vi "Main.vi"() -> ()   [LabVIEW 2016]
uses:
  VI Reference Control/VI Reference Control.lvclass
panel:
  in  "Execute Script":bool
  in  "Target Path":path
  out "Target Picture":picture
  in  "Source Path":path
  out "Source Picture":picture
  in  "stop":bool
  # "Drag Target VI Here"
  # "Drag Source VI Here"
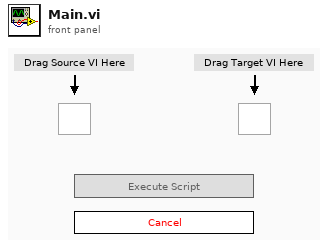
[diagram p1: front panel]
types:
  T1 = enum8{"Enabled", "Disabled", "Disabled and Grayed Out"}
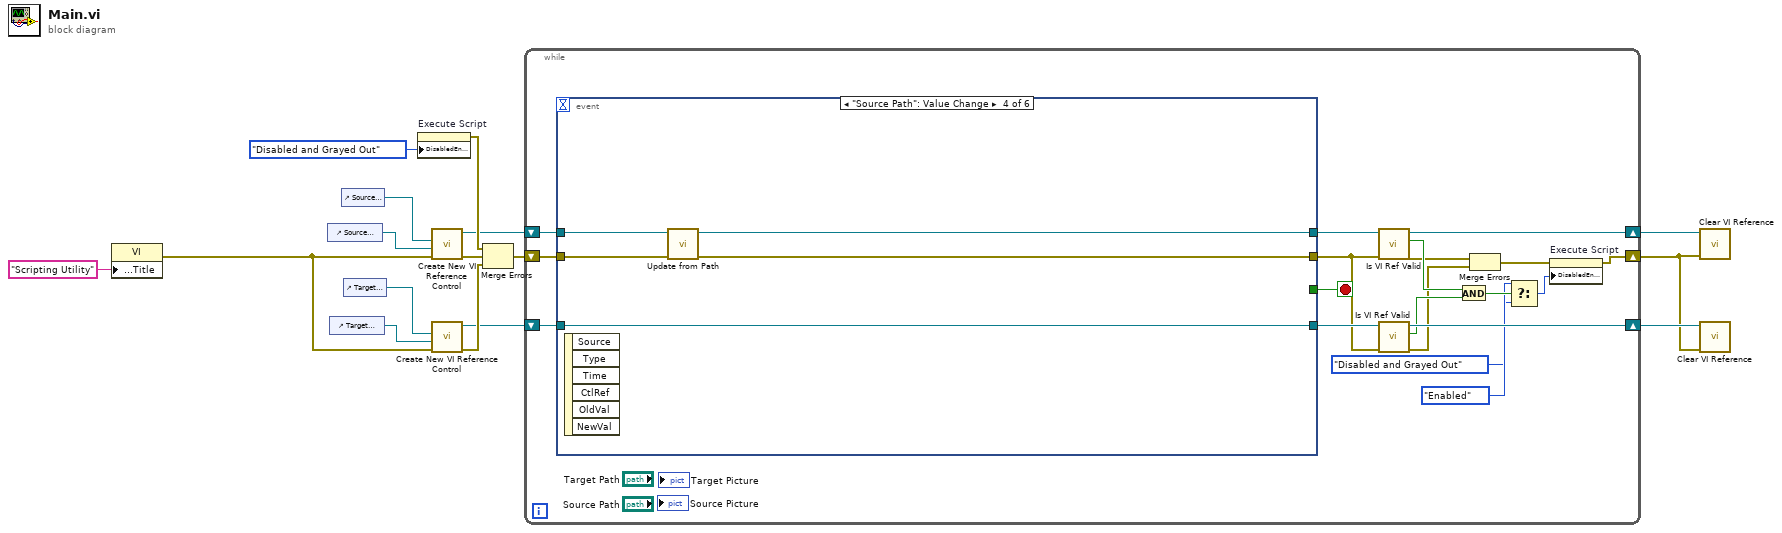
[diagram p0: block diagram]
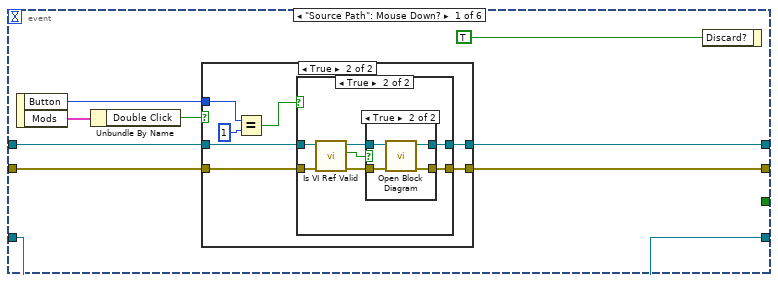
[diagram p2: hidden frame]
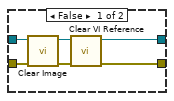
[diagram p4: hidden frame]
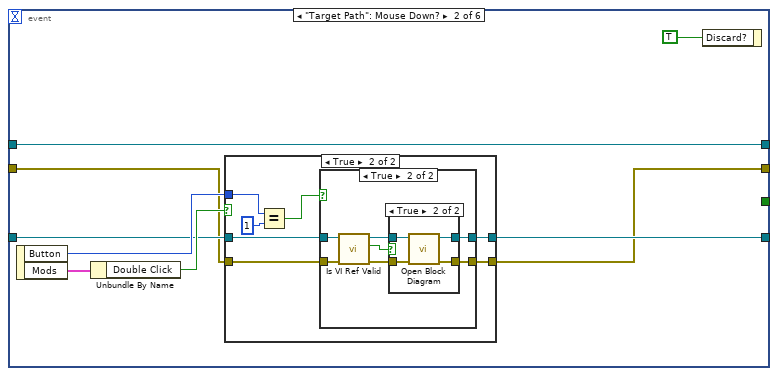
[diagram p6: hidden frame]
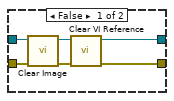
[diagram p8: hidden frame]
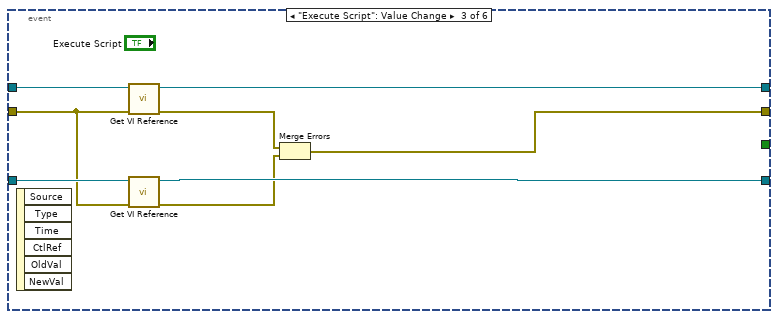
[diagram p10: hidden frame]
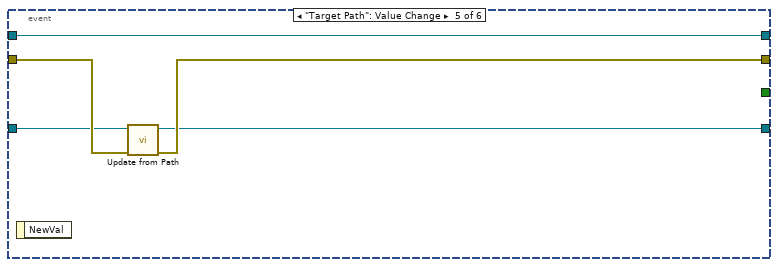
[diagram p11: hidden frame]
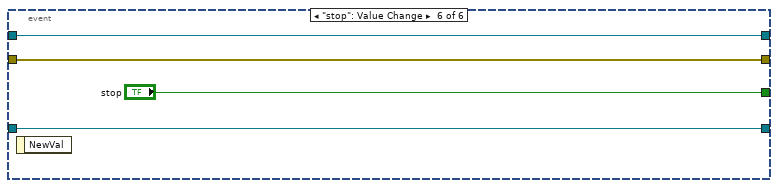
[diagram p12: hidden frame]
diagram:
  n1 = property class="VI"("Front Panel.Title"="Scripting Utility" ("Front Panel Window:Title")) -> (error out=w1:errorcluster)  [unwired: 2 in, 1 out]
  n2 = control-ref of="Source Picture"() -> (w12:refnum<vi>)
  n3 = control-ref of="Target Picture"() -> (w9:refnum<vi>)
  n4 = control-ref of="Source Path"() -> (w13:refnum<vi>)
  n5 = control-ref of="Target Path"() -> (w10:refnum<vi>)
  n6 = property on="Execute Script" class="Bool"("DisabledEnum"=T1."Disabled and Grayed Out" ("Disabled")) -> (error out=w15:errorcluster)  [unwired: 2 in, 1 out]
  n7 = call "Create New VI Reference Control.vi"("error in (no error)"=w1, "Picture Control Ref"=w12, "Path Control Ref"=w13) -> ("error out"=w8:errorcluster, "VI Reference Control out"=w11:refnum<class "VI Reference Control.lvclass">)  [unwired: 7 in]
  n8 = call "Create New VI Reference Control.vi"("error in (no error)"=w1, "Picture Control Ref"=w9, "Path Control Ref"=w10) -> ("error out"=w7:errorcluster, "VI Reference Control out"=w6:refnum<class "VI Reference Control.lvclass">)  [unwired: 7 in]
  n9 = Merge Errors(w15, w8, w7) -> (w14:errorcluster)
  n10 = while {
    shift-right: [w31] -> w3
    shift-left: w14 -> [w32]
    shift-right: [w28] -> w5
    shift-left: w11 -> [w30]
    shift-right: [w27] -> w4
    shift-left: w6 -> [w26]
    stop <- w35 stop-if-true
    n11 = event shown="[3] \"Source Path\": Value Change" {
      selector: _ -> [_ _ _ _ _ _]
      dyn-events: _ -> [_ _ _ _ _ _]
      timeout: _ -> [_ _ _ _ _ _]
      tunnel: [_ _ _ _ _ "stop"] -> w35
      tunnel: w32 -> [w40 w75 w113 w121 w127 w130]
      tunnel: [w39 w73 w110 w118 w126 w130] -> w24
      tunnel: w30 -> [w38 w79 w115 w122 w123 w129]
      tunnel: [w37 w79 w114 w120 w123 w129] -> w29
      tunnel: w26 -> [w36 w76 w117 w119 w125 w128]
      tunnel: [w36 w74 w116 w119 w124 w128] -> w25
      event "Source Path": Mouse Down? {
        n12 = event-data() -> ("Button"=w41:u16, "Mods"=w43:cluster{"Double Click":bool, "Menu Key":bool})  [unwired: 1 in]
        n13 = Unbundle By Name(w43) -> ("Double Click"=w42:bool)
        n14 = case shown="True" w42 {
          tunnel: w41 -> [_ w51]
          tunnel: w40 -> [w46 w50]
          tunnel: [w46 w49] -> w39
          tunnel: w38 -> [w45 w48]
          tunnel: [w45 w47] -> w37
          frame False {
          }
          frame True {
            n15 = Equal?(x=w51, y=u16 1) -> (x = y?=w52:bool)
            n16 = case shown="True" w52 {
              tunnel: w50 -> [w56 w61]
              tunnel: [w54 w66] -> w49
              tunnel: w48 -> [w58 w64]
              tunnel: [w59 w65] -> w47
              frame False {
                n17 = call "Clear Image.vi"("error in (no error)"=w56, "VI Reference Control in"=w58) -> ("error out"=w55:errorcluster, "VI Reference Control out"=w57:refnum<class "VI Reference Control.lvclass">)  [unwired: 8 in]
                n18 = call "Clear VI Reference.vi"("error in (no error)"=w55, "VI Reference Control in"=w57) -> ("error out"=w54:errorcluster, "VI Reference Control out"=w59:refnum<class "VI Reference Control.lvclass">)  [unwired: 8 in]
              }
              frame True {
                n19 = call "Is VI Ref Valid"("error in (no error)"=w61, "VI Reference Control in"=w64) -> ("error out"=w60:errorcluster, "Refnum Valid?"=w63:bool, "VI Reference Control out"=w62:refnum<class "VI Reference Control.lvclass">)  [unwired: 7 in]
                n20 = case shown="True" w63 {
                  tunnel: w60 -> [w68 w71]
                  tunnel: [w68 w70] -> w66
                  tunnel: w62 -> [w67 w72]
                  tunnel: [w67 w69] -> w65
                  frame False {
                  }
                  frame True {
                    n21 = call "Open Block Diagram.vi"("error in (no error)"=w71, "VI Reference Control in"=w72) -> ("error out"=w70:errorcluster, "VI Reference Control out"=w69:refnum<class "VI Reference Control.lvclass">)  [unwired: 8 in]
                  }
                }
              }
            }
          }
        }
        n22 = event-data("Discard?"=TRUE) -> ()  [unwired: 1 in, 1 out]
      }
      event "Target Path": Mouse Down? {
        n23 = event-data() -> ("Button"=w77:u16, "Mods"=w80:cluster{"Double Click":bool, "Menu Key":bool})  [unwired: 1 in]
        n24 = Unbundle By Name(w80) -> ("Double Click"=w78:bool)
        n25 = case shown="True" w78 {
          tunnel: w77 -> [_ w88]
          tunnel: w75 -> [w83 w87]
          tunnel: [w83 w86] -> w73
          tunnel: w76 -> [w82 w85]
          tunnel: [w82 w84] -> w74
          frame False {
          }
          frame True {
            n26 = Equal?(x=w88, y=u16 1) -> (x = y?=w89:bool)
            n27 = case shown="True" w89 {
              tunnel: w87 -> [w93 w98]
              tunnel: [w91 w103] -> w86
              tunnel: w85 -> [w95 w101]
              tunnel: [w96 w102] -> w84
              frame False {
                n28 = call "Clear Image.vi"("error in (no error)"=w93, "VI Reference Control in"=w95) -> ("error out"=w92:errorcluster, "VI Reference Control out"=w94:refnum<class "VI Reference Control.lvclass">)  [unwired: 8 in]
                n29 = call "Clear VI Reference.vi"("error in (no error)"=w92, "VI Reference Control in"=w94) -> ("error out"=w91:errorcluster, "VI Reference Control out"=w96:refnum<class "VI Reference Control.lvclass">)  [unwired: 8 in]
              }
              frame True {
                n30 = call "Is VI Ref Valid"("error in (no error)"=w98, "VI Reference Control in"=w101) -> ("error out"=w97:errorcluster, "Refnum Valid?"=w100:bool, "VI Reference Control out"=w99:refnum<class "VI Reference Control.lvclass">)  [unwired: 7 in]
                n31 = case shown="True" w100 {
                  tunnel: w97 -> [w105 w108]
                  tunnel: [w105 w107] -> w103
                  tunnel: w99 -> [w104 w109]
                  tunnel: [w104 w106] -> w102
                  frame False {
                  }
                  frame True {
                    n32 = call "Open Block Diagram.vi"("error in (no error)"=w108, "VI Reference Control in"=w109) -> ("error out"=w107:errorcluster, "VI Reference Control out"=w106:refnum<class "VI Reference Control.lvclass">)  [unwired: 8 in]
                  }
                }
              }
            }
          }
        }
        n33 = event-data("Discard?"=TRUE) -> ()  [unwired: 1 in, 1 out]
      }
      event "Execute Script": Value Change {
        n34 = event-data() -> ()  [unwired: 1 in, 6 out]
        n35 = call "Get VI Reference.vi"("error in (no error)"=w113, "VI Reference Control in"=w115) -> ("error out"=w112:errorcluster, "VI Reference Control out"=w114:refnum<class "VI Reference Control.lvclass">)  [unwired: 7 in, 1 out]
        n36 = call "Get VI Reference.vi"("error in (no error)"=w113, "VI Reference Control in"=w117) -> ("error out"=w111:errorcluster, "VI Reference Control out"=w116:refnum<class "VI Reference Control.lvclass">)  [unwired: 7 in, 1 out]
        n37 = Merge Errors(w112, w111) -> (w110:errorcluster)
      }
      event "Source Path": Value Change {
        n38 = event-data() -> ()  [unwired: 1 in, 6 out]
        n39 = call "Update from Path.vi"("error in (no error)"=w121, "VI Reference Control in"=w122) -> ("error out"=w118:errorcluster, "VI Reference Control out"=w120:refnum<class "VI Reference Control.lvclass">)  [unwired: 8 in]
      }
      event "Target Path": Value Change {
        n40 = event-data() -> ()  [unwired: 1 in, 1 out]
        n41 = call "Update from Path.vi"("error in (no error)"=w127, "VI Reference Control in"=w125) -> ("error out"=w126:errorcluster, "VI Reference Control out"=w124:refnum<class "VI Reference Control.lvclass">)  [unwired: 8 in]
      }
      event "stop": Value Change {
        n42 = event-data() -> ()  [unwired: 1 in, 1 out]
      }
    }
    n43 = call "Is VI Ref Valid"("error in (no error)"=w24, "VI Reference Control in"=w29) -> ("error out"=w21:errorcluster, "Refnum Valid?"=w22:bool, "VI Reference Control out"=w28:refnum<class "VI Reference Control.lvclass">)  [unwired: 7 in]
    n44 = call "Is VI Ref Valid"("error in (no error)"=w24, "VI Reference Control in"=w25) -> ("error out"=w20:errorcluster, "Refnum Valid?"=w23:bool, "VI Reference Control out"=w27:refnum<class "VI Reference Control.lvclass">)  [unwired: 7 in]
    n45 = And(x=w22, y=w23) -> (x .and. y?=w34:bool)
    n46 = Merge Errors(w21, w20) -> (w19:errorcluster)
    n47 = Select(t=T1."Enabled" ("f"), s=w34, f=T1."Disabled and Grayed Out" ("Disabled")) -> (s? t:f=w33:T1)
    n48 = property on="Execute Script" class="Bool"(error in=w19, "DisabledEnum"=w33) -> (error out=w31:errorcluster)  [unwired: 1 in, 1 out]
  }
  n49 = call "Clear VI Reference.vi"("error in (no error)"=w3, "VI Reference Control in"=w5) -> ()  [unwired: 8 in, 2 out]
  n50 = call "Clear VI Reference.vi"("error in (no error)"=w3, "VI Reference Control in"=w4) -> ()  [unwired: 8 in, 2 out]
